vi "monitor.vi"(11 "Command":string) -> ()   [LabVIEW 2018, in "SyncModule.lvlib"]
uses:
  SyncModule.lvlib
panel:
  in  "Clear":bool
  out "Commands":string
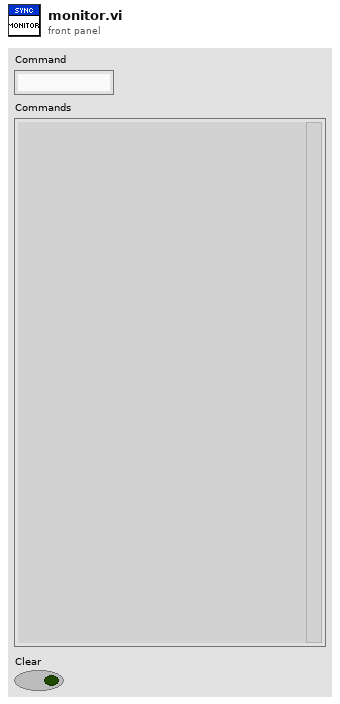
[diagram p1: front panel]
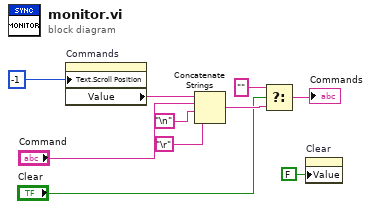
[diagram p0: block diagram]
diagram:
  n1 = property on="Commands" class="Str"("Text.Scroll Position"=-1) -> ("Value"=w9:string)  [unwired: 2 in, 2 out]
  n2 = Concatenate Strings(w9, "Command", "\n", "\r") -> (w4:string)
  n3 = Select(t="", s="Clear", f=w4) -> (s? t:f=→"Commands":string)
  n4 = property on="Clear" class="Bool (strict)"("Value"=FALSE ("Clear")) -> ()  [unwired: 2 in, 2 out]
